vi "Measurement Type to Channel Info.vi"(10 "Measurement Type":T2) -> (1 "channel classification":T3, 3 "Data Type":T1)   [LabVIEW 2014, in "DAQmx Module Editor Node.lvclass"]
doc: "Converts from the 'display permissions' type-def to the 'channel classification' type-def."
uses:
  DAQmx Module Editor Node.lvclass
  <vilib>/NI/Tag Bus Module Framework/channel/channel classification.ctl
  module/configuration/Measurement Type.ctl
  <vilib>/NI/Tag Bus/tag/Data Type.ctl
  <vilib>/NI/Tag Bus Module Framework/channel/TBM channel.lvclass
  <vilib>/NI/Tag Bus/tag/tag descriptor.lvclass
  module/configuration/DAQmx Module Configuration.lvclass
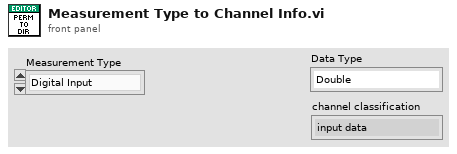
[diagram p1: front panel]
types:
  T1 = typedef "tag bus.lvlib/tag descriptor.lvclass/Data Type.ctl" = enum16{"Double", "Single", "I64", "I32", "I16", "I8", "U64", "U32", "U16", "U8", "Boolean", "String", "Array of Double", "Array of Single", "Array of I64", "Array of I32", "Array of I16", "Array of I8", "Array of U64", "Array of U32", "Array of U16", "Array of U8", "Array of Boolean", "Array of String"}
  T2 = typedef "DAQmx Module Configuration.lvclass/Measurement Type.ctl" = enum16{"Digital Input", "Digital Output", "Voltage Input", "Voltage Output", "Current Input", "Current Output", "RTD", "Thermocouple", "Strain"}
  T3 = typedef "TBM channel.lvclass/channel classification.ctl" = enum16{"input data", "output data", "processing parameter", "processing result"}
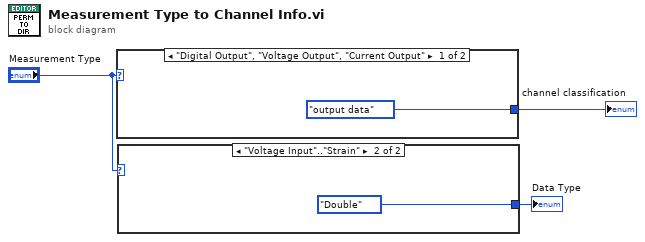
[diagram p0: block diagram]
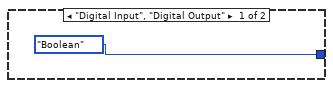
[diagram p2: hidden frame]
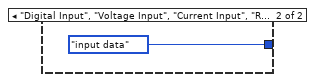
[diagram p3: hidden frame]
diagram:
  n1 = case shown="\"Digital Output\", \"Voltage Output\", \"Current Output\"" "Measurement Type" {
    tunnel: [channel_classification."output data" ("channel classification") channel_classification."input data" ("channel classification")] -> w3
    frame "Digital Output", "Voltage Output", "Current Output" {
    }
    frame "Digital Input", "Voltage Input", "Current Input", "RTD".."Strain" {
    }
  }
  "channel classification" <- w3
  n2 = case shown="\"Voltage Input\"..\"Strain\"" "Measurement Type" {
    tunnel: [Data_Type."Boolean" ("Data Type") Data_Type."Double" ("Data Type")] -> w1
    frame "Digital Input", "Digital Output" {
    }
    frame "Voltage Input".."Strain" {
    }
  }
  "Data Type" <- w1
